vi "_convert_string_to_time.vi"(8 "error in (no error)":errorcluster, 11 "Input string":string) -> (0 "error out":errorcluster, 2 "Time String":string, 3 "Time in seconds":dbl)   [LabVIEW 2016, in "Chemyx_Syringe_Pump_driver.lvlib"]
doc: "Converts the input string representing time in hours into a string in the format \"X hr YY min ZZ sec\"."
uses:
  Chemyx_Syringe_Pump_driver.lvlib
panel:
  # "#Description\nConverts the input string representing time in hours into a string in the format \"X hr YY min ZZ sec\"."
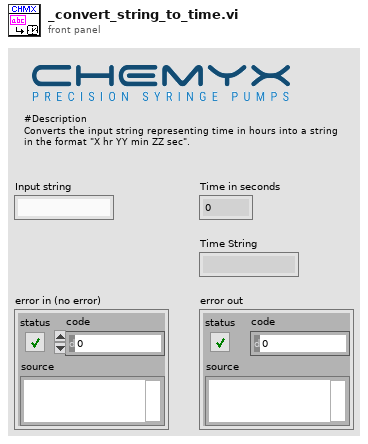
[diagram p1: front panel]
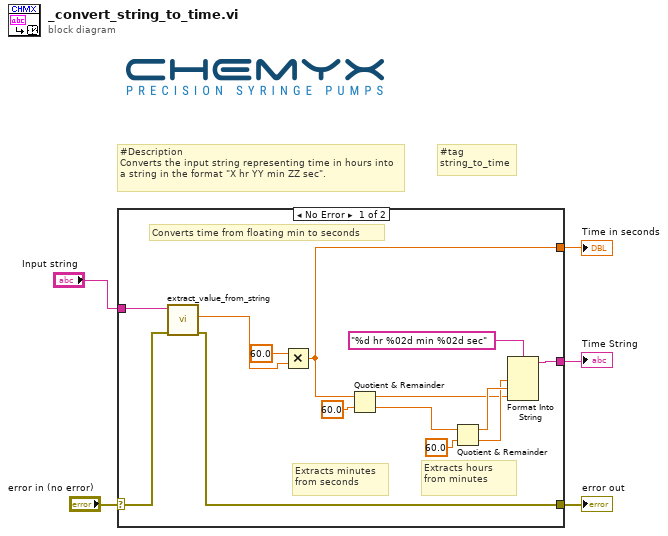
[diagram p0: block diagram]
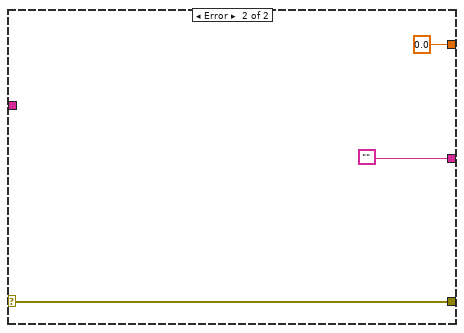
[diagram p2: hidden frame]
diagram:
  # "#tag\nstring_to_time"
  # "#Description\nConverts the input string representing time in hours into a string in the format \"X hr YY min ZZ sec\"."
  n1 = case shown="No Error" "error in (no error)" {
    selector: "error in (no error)" -> [w9 w21]
    tunnel: [w19 ""] -> w5
    tunnel: [w18 0.0] -> w4
    tunnel: "Input string" -> [w11 _]
    tunnel: [w10 w21] -> w2
    frame No Error {
      # "Extracts hours from minutes"
      # "Extracts minutes from seconds"
      # "Converts time from floating min to seconds"
      n2 = call "extract_value_from_string.vi"("error in (no error)"=w9, "Input string"=w11) -> ("error out"=w10:errorcluster, "Value"=w8:dbl)  [unwired: 7 in, 1 out]
      n3 = Multiply(x=60.0, y=w8) -> (x*y=w18:dbl)
      n4 = Quotient & Remainder(x=w18, y=60.0 ("x")) -> (x-y*floor(x/y)=w13:dbl, floor(x/y)=w14:dbl)
      n5 = Quotient & Remainder(x=w14, y=60.0 ("x")) -> (x-y*floor(x/y)=w17:dbl, floor(x/y)=w16:dbl)
      n6 = Format Into String(format string="%d hr %02d min %02d sec", w16, w17, w13) -> (resulting string=w19:string)  [unwired: 2 in, 1 out]
    }
    frame Error {
    }
  }
  "Time String" <- w5
  "Time in seconds" <- w4
  "error out" <- w2
